vi "Write Configuration.vi"(8 "error in (no error)":errorcluster, 11 "Error Handler In":refnum<class "Error Handler.lvclass">) -> (0 "error out":errorcluster, 3 "Error Handler Out":refnum<class "Error Handler.lvclass">)   [LabVIEW 2020, in "Error Handler.lvclass"]
doc: "Method that write the object attributes to config file."
uses:
  Error Handler.lvclass
  Support/Configuration File/Configuration File.lvlib
  Process/Process.lvclass
  Support/Error Log Classes/Error Log/Error Log.lvclass
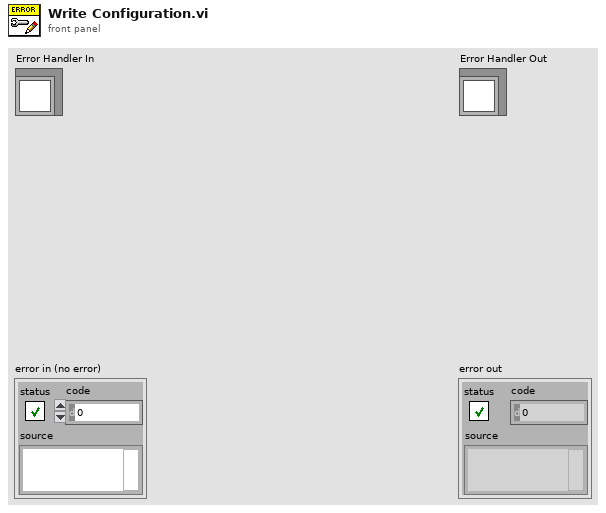
[diagram p1: front panel]
types:
  T1 = typedef "NI_LVConfig.lvlib/Config Data RefNum.ctl" = refnum<k1>
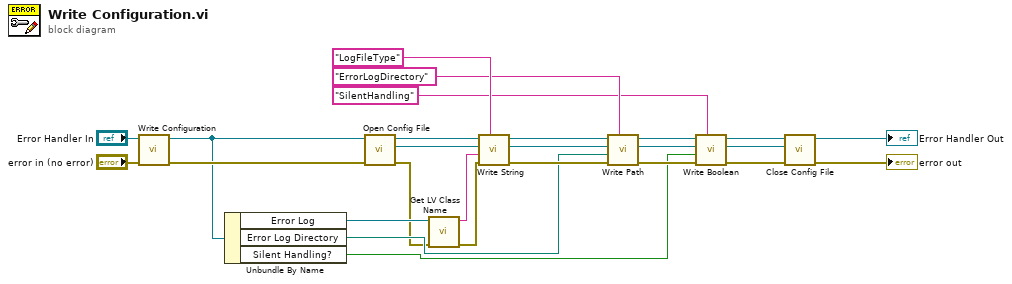
[diagram p0: block diagram]
diagram:
  n1 = call-parent "Write Configuration.vi"("error in (no error)"="error in (no error)", "Process In"="Error Handler In") -> ("error out"=w21:errorcluster, "Process Out"=w7:refnum<class "Error Handler.lvclass">)  [unwired: 8 in]
  n2 = Unbundle By Name(w7) -> ("Error Log"=w6:refnum<class "Error Log.lvclass">, "Error Log Directory"=w4:path, "Silent Handling?"=w3:bool)
  n3 = call "Open Config File.vi"("error in (no error)"=w21, "Process in"=w7) -> ("error out"=w1:errorcluster, "refnum out"=w15:T1, "Process out"=w22:refnum<class "Error Handler.lvclass">)  [unwired: 6 in, 1 out]
  n4 = call <vilib>:"Get LV Class Name.vi"("error in (no error)"=w1, "object"=w6) -> ("error out"=w2:errorcluster, "class name"=w5:string)  [unwired: 8 in]
  n5 = call "Write String.vi"("key"="LogFileType", "error in (no error)"=w2, "default value"=w5, "refnum"=w15, "Process in"=w22) -> ("error out"=w13:errorcluster, "refnum out"=w14:T1, "Process out"=w24:refnum<class "Error Handler.lvclass">)  [unwired: 4 in]
  n6 = call "Write Path.vi"("key"="ErrorLogDirectory", "error in (no error)"=w13, "default value"=w4, "refnum"=w14, "Process in"=w24) -> ("error out"=w11:errorcluster, "refnum out"=w12:T1, "Process out"=w19:refnum<class "Error Handler.lvclass">)  [unwired: 4 in]
  n7 = call "Write Boolean.vi"("key"="SilentHandling", "error in (no error)"=w11, "default value"=w3, "refnum"=w12, "Process in"=w19) -> ("error out"=w9:errorcluster, "refnum out"=w10:T1, "Process out"=w17:refnum<class "Error Handler.lvclass">)  [unwired: 4 in]
  n8 = call "Close Config File.vi"("error in (no error)"=w9, "refnum"=w10, "Process in"=w17) -> ("error out"=→"error out":errorcluster, "Process out"=→"Error Handler Out":refnum<class "Error Handler.lvclass">)  [unwired: 6 in, 1 out]
